vi "Read Panel Resized.vi"(11 "Flex  Dialog (Actor) in":refnum<class "Flex Dialog (Actor).lvclass">) -> (2 "Panel Resized":refnum<class "MVC Subscription.lvclass">, 3 "Flex  Dialog (Actor) out":refnum<class "Flex Dialog (Actor).lvclass">)   [LabVIEW 2014, in "Flex UI Dialog (Actor).lvlib" / "Flex Dialog (Actor).lvclass"]
uses:
  Flex Dialog (Actor).lvclass
  <vilib>/East West Architects/MVC Subscription/Subscription/MVC Subscription.lvclass
  Flex Dialog (Actor).lvclass/Flex Dialog (Actor).ctl
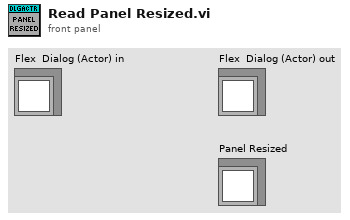
[diagram p1: front panel]
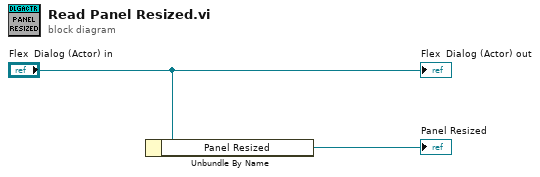
[diagram p0: block diagram]
diagram:
  n1 = Unbundle By Name("Flex  Dialog (Actor) in") -> ("Panel Resized"=→"Panel Resized":refnum<class "MVC Subscription.lvclass">)
  "Flex  Dialog (Actor) out" <- "Flex  Dialog (Actor) in"
